vi "Edit-settings.vi"(8 "error in (no error)":errorcluster, 11 "HC-LaserPulse in":refnum<class "HC-LaserResponse.lvclass">) -> (0 "error out":errorcluster, 3 "HC-LaserPulse out":refnum<class "HC-LaserResponse.lvclass">)   [LabVIEW 2013, in "HardwareCharacterization.lvlib" / "HC-LaserResponse.lvclass"]
doc: "Use this template to build a VI to use as a subVI."
uses:
  HC-LaserResponse.lvclass
  Settings.ctl
  Settings-storage.ctl
  Settings-zero.ctl
  Settings-stable.ctl
  Settings-divide.ctl
  Settings-reaction.ctl
  Settings-response.ctl
  Settings-stabilization.ctl
  Settings-shutdown.ctl
  Settings-extinction.ctl
  Test-characteristics.ctl
  Detectors.ctl
  HC-LaserResponse.lvclass/HC-LaserResponse.ctl
panel:
  in  "Test characteristics":T1={"Record length"=0, "Time interval [s]"=5e-06, "Note"="", "Laser control mode"=enum."Modulation (digital)", "Power [Watt]"=0.0, "Power [%]"=0.0, "Pulse rate [Hz]"=0.0, "Detector"=enum."DET10A - 2kOhm ", "Duty cycle [%]"=50.0}
  in  "Cancel":bool
  in  "Ok":bool
  in  "Pulse analysis settings":T3={"Storage settings"={"Group results"=FALSE, "Append/overwrite"=FALSE}, "Zero level settings"={"Lower fraction [%]"=10, "Max. delta [Volt]"=0.5, "Min. segment length"=100}, "Stable level settings"={"Top fraction [%]"=10, "Max. delta [Volt]"=0.5, "Min. segment length"=100}, "Sample divide settings"={"Accept only complete pulses"=TRUE, "Edge treshold [%]"=15}, "Reaction time settings"={"Treshold [%]"=15}, "Response time settings"={"Treshold [%]"=85}, "Stabilization time settings"={"Max. delta [%]"=15, "Min. segment length"=50}, "Shutdown time settings"={"Treshold [%]"=85}, "Extinction time settings"={"Treshold [%]"=15}, "Spike detection settings"={"Treshold [%]"=30}}
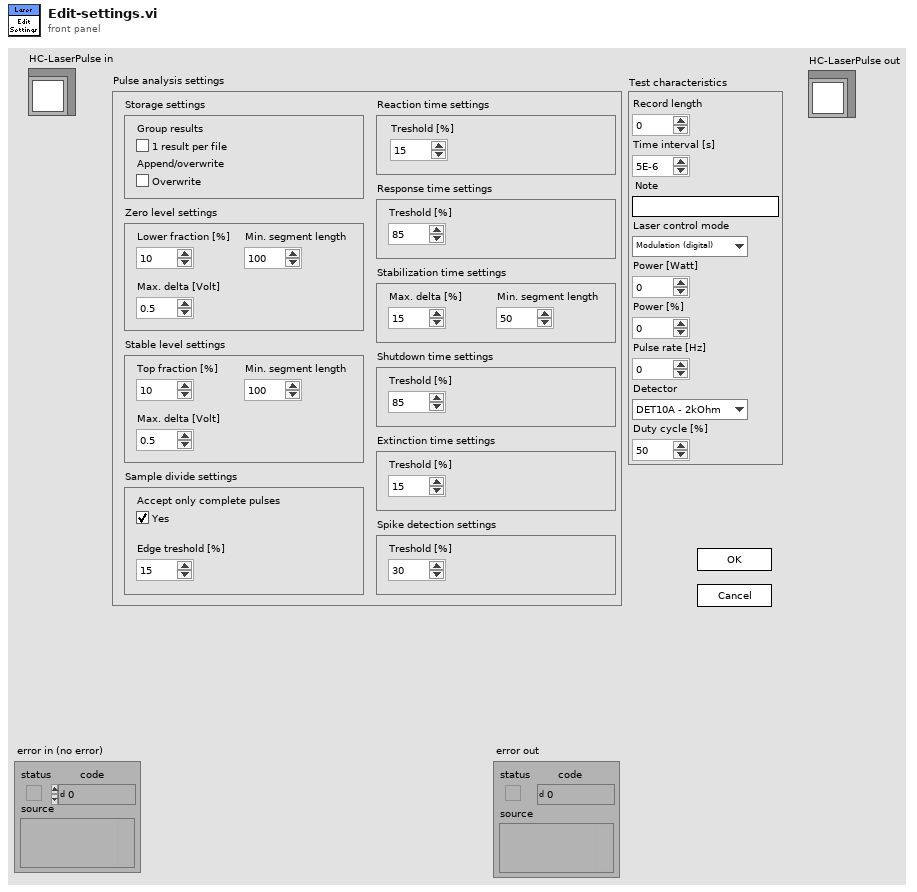
[diagram p1: front panel]
types:
  T1 = typedef "HardwareCharacterization.lvlib/HC-LaserResponse.lvclass/Test-characteristics.ctl" = cluster{"Record length":i32, "Time interval [s]":dbl, "Note":string, "Laser control mode":enum16{"Undefined", "Modulation (digital)", "Power variation (analog)"}, "Power [Watt]":dbl, "Power [%]":dbl, "Pulse rate [Hz]":dbl, "Detector":T2, "Duty cycle [%]":dbl}
  T2 = typedef "HardwareCharacterization.lvlib/HC-LaserResponse.lvclass/Detectors.ctl" = enum16{"Undefined", "DET10A", "DET10A - 2kOhm ", "PDA36A - 0dB"}
  T3 = typedef "HardwareCharacterization.lvlib/HC-LaserResponse.lvclass/Settings.ctl" = cluster{"Storage settings":T4, "Zero level settings":T5, "Stable level settings":T6, "Sample divide settings":T7, "Reaction time settings":T8, "Response time settings":T9, "Stabilization time settings":T10, "Shutdown time settings":T11, "Extinction time settings":T12, "Spike detection settings":cluster{"Treshold [%]":i32}}
  T4 = typedef "HardwareCharacterization.lvlib/HC-LaserResponse.lvclass/Settings-storage.ctl" = cluster{"Group results":bool, "Append/overwrite":bool}
  T5 = typedef "HardwareCharacterization.lvlib/HC-LaserResponse.lvclass/Settings-zero.ctl" = cluster{"Lower fraction [%]":i32, "Max. delta [Volt]":dbl, "Min. segment length":i32}
  T6 = typedef "HardwareCharacterization.lvlib/HC-LaserResponse.lvclass/Settings-stable.ctl" = cluster{"Top fraction [%]":i32, "Max. delta [Volt]":dbl, "Min. segment length":i32}
  T7 = typedef "HardwareCharacterization.lvlib/HC-LaserResponse.lvclass/Settings-divide.ctl" = cluster{"Accept only complete pulses":bool, "Edge treshold [%]":i32}
  T8 = typedef "HardwareCharacterization.lvlib/HC-LaserResponse.lvclass/Settings-reaction.ctl" = cluster{"Treshold [%]":i32}
  T9 = typedef "HardwareCharacterization.lvlib/HC-LaserResponse.lvclass/Settings-response.ctl" = cluster{"Treshold [%]":i32}
  T10 = typedef "HardwareCharacterization.lvlib/HC-LaserResponse.lvclass/Settings-stabilization.ctl" = cluster{"Max. delta [%]":i32, "Min. segment length":i32}
  T11 = typedef "HardwareCharacterization.lvlib/HC-LaserResponse.lvclass/Settings-shutdown.ctl" = cluster{"Treshold [%]":i32}
  T12 = typedef "HardwareCharacterization.lvlib/HC-LaserResponse.lvclass/Settings-extinction.ctl" = cluster{"Treshold [%]":i32}
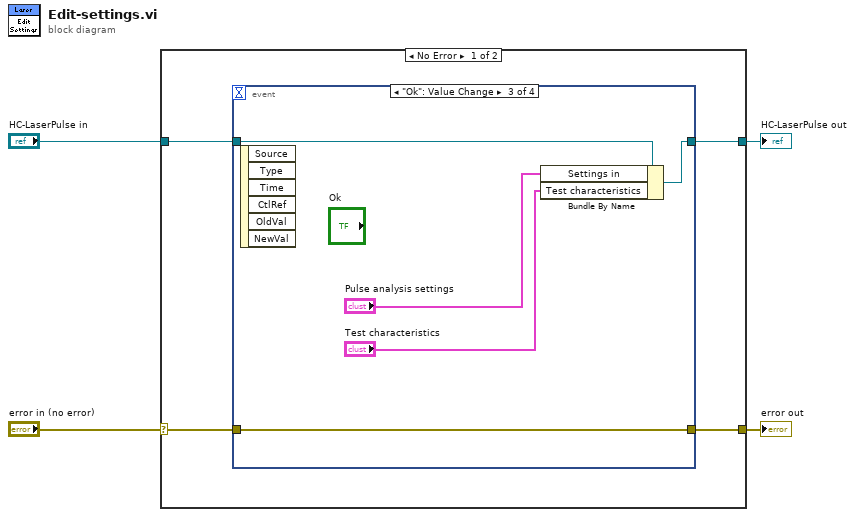
[diagram p0: block diagram]
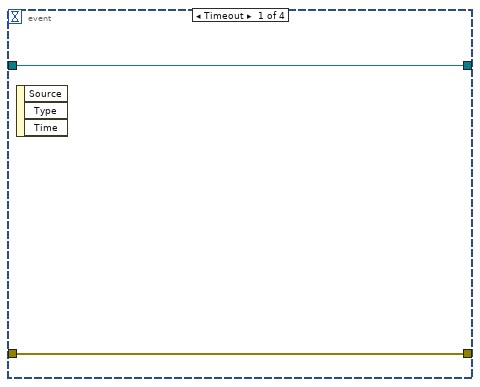
[diagram p2: hidden frame]
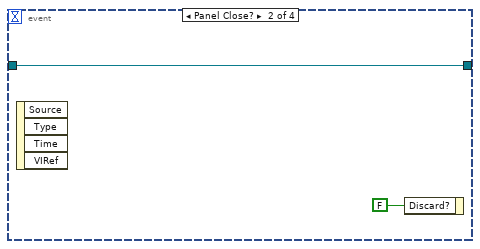
[diagram p3: hidden frame]
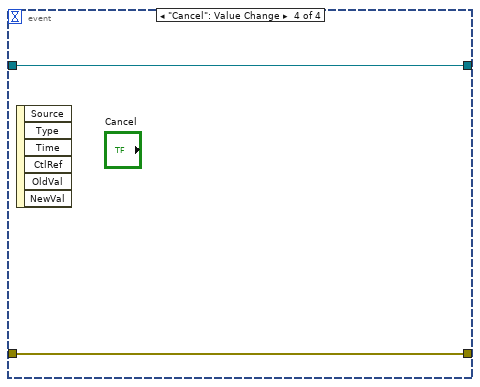
[diagram p4: hidden frame]
diagram:
  n1 = case shown="No Error" "error in (no error)" {
    selector: "error in (no error)" -> [w8 w21]
    tunnel: [w7 w21] -> w3
    tunnel: "HC-LaserPulse in" -> [w6 w20]
    tunnel: [w5 w20] -> w1
    frame No Error {
      n2 = event shown="[2] \"Ok\": Value Change" {
        selector: _ -> [_ _ _ _]
        dyn-events: _ -> [_ _ _ _]
        timeout: _ -> [_ _ _ _]
        tunnel: w8 -> [w10 _ w17 w19]
        tunnel: [w10 _ w17 w19] -> w7
        tunnel: w6 -> [w9 w11 w16 w18]
        tunnel: [w9 w11 w15 w18] -> w5
        event Timeout {
          n3 = event-data() -> ()  [unwired: 1 in, 3 out]
        }
        event Panel Close? {
          n4 = event-data() -> ()  [unwired: 1 in, 4 out]
          n5 = event-data("Discard?"=FALSE) -> ()  [unwired: 1 in, 1 out]
        }
        event "Ok": Value Change {
          n6 = event-data() -> ()  [unwired: 1 in, 6 out]
          n7 = Bundle By Name(cluster=w16, "Settings in"="Pulse analysis settings", "Test characteristics"="Test characteristics") -> (w15:refnum<class "HC-LaserResponse.lvclass">)
        }
        event "Cancel": Value Change {
          n8 = event-data() -> ()  [unwired: 1 in, 6 out]
        }
      }
    }
    frame Error {
    }
  }
  "error out" <- w3
  "HC-LaserPulse out" <- w1
